vi "create.AddOrderLong.vi"(11 "AddOrderLong.Parameters":T1={"Time Offset"=447000, "Order Id"="ORID0001", "Quantity"=20000, "Symbol"="AAPL", "Side Indicator"="B", "Price"=0.905}) -> (2 "Bytes.Out":u8[](array[numeric])=[34, 33, 24, 210, 6, 0, 79, 82, 73, 68, 48, 48, 48, 49, 66, 32, 78, 0, 0, 65, 65, 80, 76, 32, 32, 90, 35, 0, 0, 0, 0, 0, 0, 1] format="%.0x", 3 "MessageBase out":refnum<class "MessageBase.lvclass">)   [LabVIEW 2020]
uses:
  AddOrder/AddOrderLong.Parameters.ctl
  MessageBase/MessageBase.lvclass
  AddOrder/AddOrderLong.lvclass
  C:/work/fpganow/Market.Data.PoC/submodules/Market.Data.Bats.Parser/host/pitch/MessageBase/MessageBase.lvclass
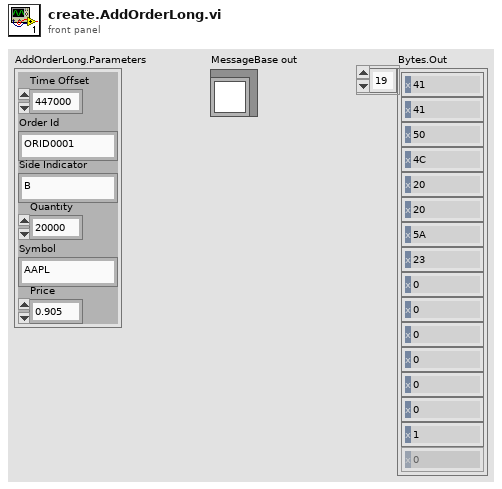
[diagram p1: front panel]
types:
  T1 = typedef "AddOrderLong.lvclass/AddOrderLong.Parameters.ctl" = cluster{"Time Offset":u32, "Order Id":string, "Quantity":u32, "Symbol":string, "Side Indicator":string, "Price":dbl}
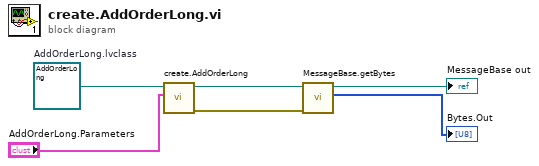
[diagram p0: block diagram]
diagram:
  w2 = refnum<class "AddOrderLong.lvclass"> refnum  # AddOrderLong.lvclass
  n1 = call-dynamic "create.AddOrderLong.vi"("AddOrderLong.Parameters"="AddOrderLong.Parameters", "AddOrderLong in"=w2) -> ("error out"=w6:errorcluster, "AddOrderLong out"=w1:refnum<class "AddOrderLong.lvclass">)  [unwired: 8 in]
  n2 = call-dynamic "MessageBase.getBytes.vi"("error in (no error)"=w6, "MessageBase in"=w1) -> ("Bytes.out"=→"Bytes.Out":u8[], "MessageBase out"=→"MessageBase out":refnum<class "AddOrderLong.lvclass">)  [unwired: 7 in, 1 out]
